vi "Result FGV.vi"(6 "Action(Get All Data)":T2=enum."Get All Data", 8 "error in":errorcluster, 11 "Result FGV Data In":T1) -> (0 "error out":errorcluster, 3 "Result FGV Data Out":T1)   [LabVIEW 2023, in "HardwareAbstractionLayer_LVOOP.lvlib" / "Report.lvclass"]
uses:
  Report.lvclass
  Control/Action FGV.ctl
  Control/Result FGV Data.ctl
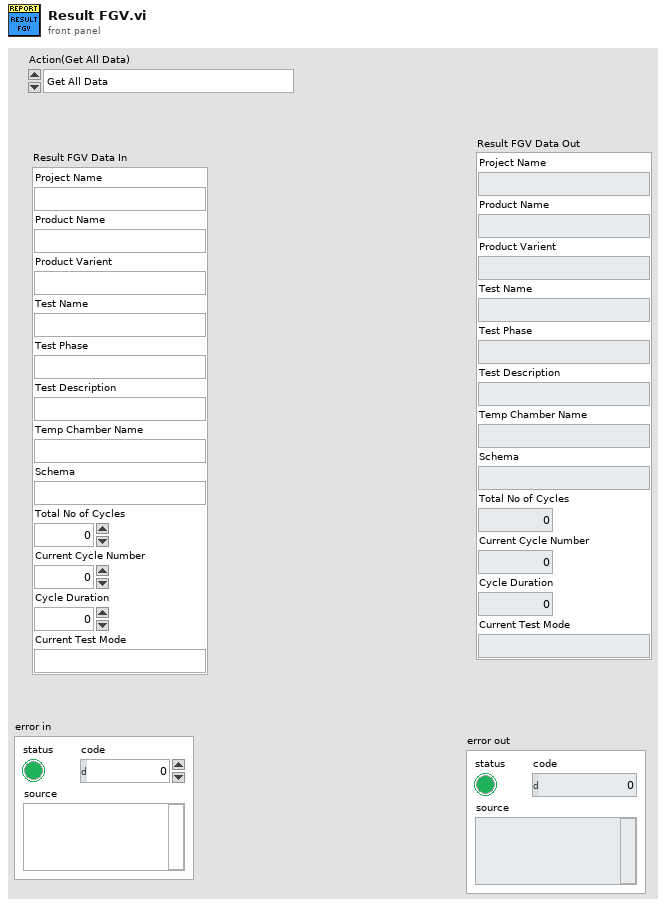
[diagram p1: front panel]
types:
  T1 = typedef "HardwareAbstractionLayer_LVOOP.lvlib/Report.lvclass/Result FGV Data.ctl" = cluster{"Project Name":string, "Product Name":string, "Product Varient":string, "Test Name":string, "Test Phase":string, "Test Description":string, "Temp Chamber Name":string, "Schema":string, "Total No of Cycles":u32, "Current Cycle Number":u32, "Cycle Duration":u32, "Current Test Mode":string}
  T2 = typedef "HardwareAbstractionLayer_LVOOP.lvlib/Report.lvclass/Action FGV.ctl" = enum16{"Init", "Set Project Name", "Set Product Name", "Set Product Varient", "Set Test Name", "Set Test Phase", "Set Test Description", "Set Temp Chamber Name", "Set Cycle Duration", "Set Current Cycle Number", "Set Schema", "Set Total No Of Cycle", "Set Current Test Mode", "Set All Data", "Get All Data"}
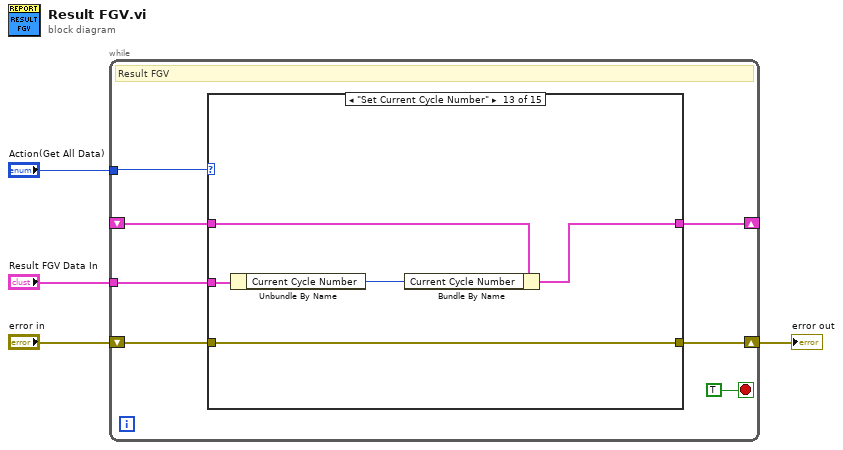
[diagram p0: block diagram]
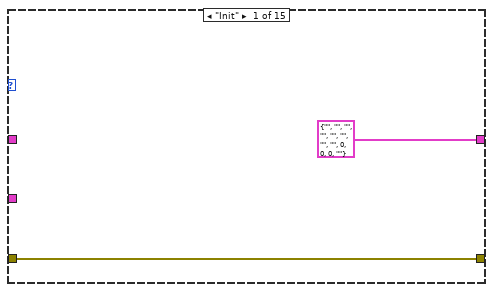
[diagram p2: hidden frame]
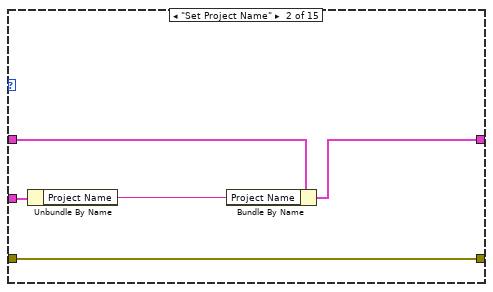
[diagram p3: hidden frame]
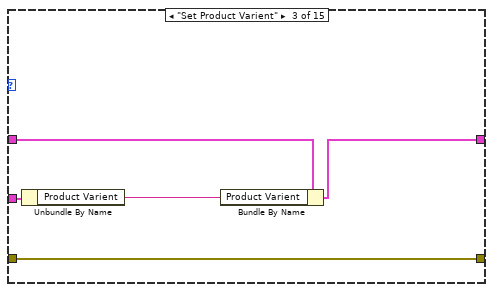
[diagram p4: hidden frame]
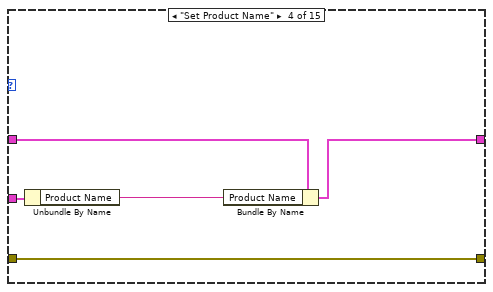
[diagram p5: hidden frame]
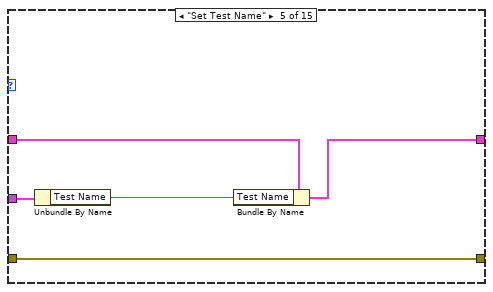
[diagram p6: hidden frame]
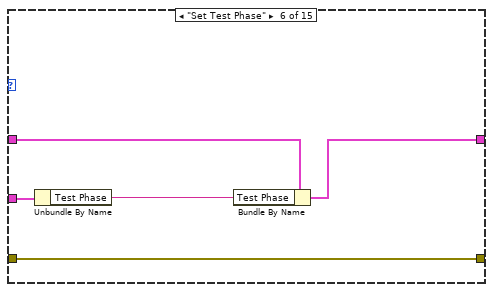
[diagram p7: hidden frame]
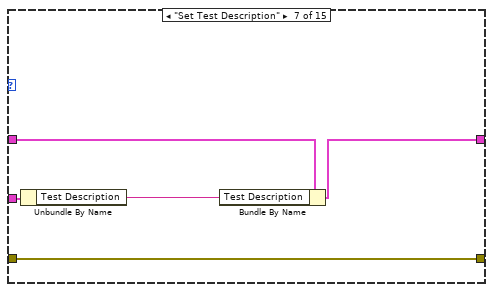
[diagram p8: hidden frame]
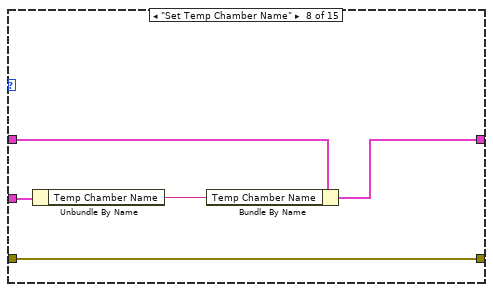
[diagram p9: hidden frame]
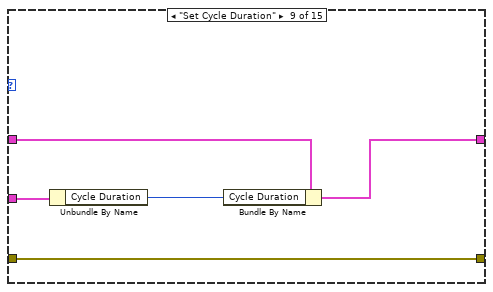
[diagram p10: hidden frame]
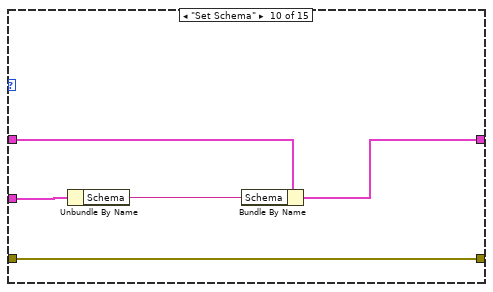
[diagram p11: hidden frame]
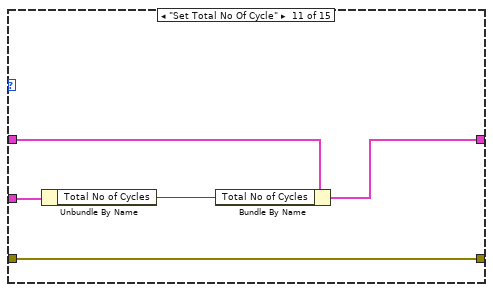
[diagram p12: hidden frame]
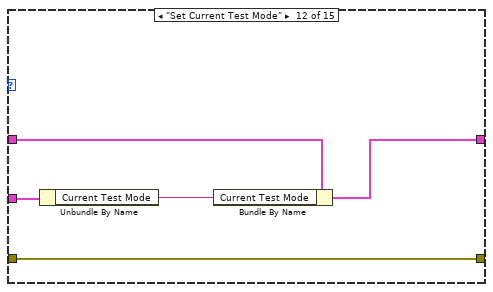
[diagram p13: hidden frame]
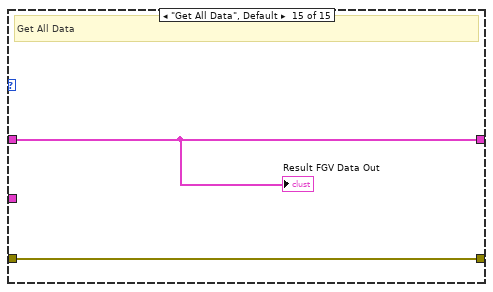
[diagram p15: hidden frame]
diagram:
  n1 = while {
    tunnel: "Action(Get All Data)" -> [w10]
    shift-right: [w8] -> w2
    shift-left: "error in" -> [w9]
    shift-right: [w6] -> _
    shift-left: _ -> [w7]
    tunnel: "Result FGV Data In" -> [w5]
    stop <- TRUE stop-if-true
    # "Result FGV"
    n2 = case shown="\"Set Current Cycle Number\"" w10 {
      tunnel: w9 -> [w13 w18 w23 w28 w33 w38 w43 w48 w53 w58 w63 w68 w73 w75 w77]
      tunnel: [w13 w18 w23 w28 w33 w38 w43 w48 w53 w58 w63 w68 w73 w75 w77] -> w8
      tunnel: w7 -> [_ w17 w22 w27 w32 w37 w42 w47 w52 w57 w62 w67 w72 _ w76]
      tunnel: [T1 {"Project Name"="", "Product Name"="", "Product Varient"="", "Test Name"="", "Test Phase"="", "Test Description"="", "Temp Chamber Name"="", "Schema"="", "Total No of Cycles"=0, "Current Cycle Number"=0, "Cycle Duration"=0, "Current Test Mode"=""} ("Result FGV Data") w16 w21 w26 w31 w36 w41 w46 w51 w56 w61 w66 w71 w74 w76] -> w6
      tunnel: w5 -> [_ w15 w20 w25 w30 w35 w40 w45 w50 w55 w60 w65 w70 w74 _]
      frame "Init" {
      }
      frame "Set Project Name" {
        n3 = Unbundle By Name(w15) -> ("Project Name"=w14:string)
        n4 = Bundle By Name(cluster=w17, "Project Name"=w14) -> (w16:T1)
      }
      frame "Set Product Varient" {
        n5 = Unbundle By Name(w20) -> ("Product Varient"=w19:string)
        n6 = Bundle By Name(cluster=w22, "Product Varient"=w19) -> (w21:T1)
      }
      frame "Set Product Name" {
        n7 = Unbundle By Name(w25) -> ("Product Name"=w24:string)
        n8 = Bundle By Name(cluster=w27, "Product Name"=w24) -> (w26:T1)
      }
      frame "Set Test Name" {
        n9 = Unbundle By Name(w30) -> ("Test Name"=w29:string)
        n10 = Bundle By Name(cluster=w32, "Test Name"=w29) -> (w31:T1)
      }
      frame "Set Test Phase" {
        n11 = Unbundle By Name(w35) -> ("Test Phase"=w34:string)
        n12 = Bundle By Name(cluster=w37, "Test Phase"=w34) -> (w36:T1)
      }
      frame "Set Test Description" {
        n13 = Unbundle By Name(w40) -> ("Test Description"=w39:string)
        n14 = Bundle By Name(cluster=w42, "Test Description"=w39) -> (w41:T1)
      }
      frame "Set Temp Chamber Name" {
        n15 = Unbundle By Name(w45) -> ("Temp Chamber Name"=w44:string)
        n16 = Bundle By Name(cluster=w47, "Temp Chamber Name"=w44) -> (w46:T1)
      }
      frame "Set Cycle Duration" {
        n17 = Unbundle By Name(w50) -> ("Cycle Duration"=w49:u32)
        n18 = Bundle By Name(cluster=w52, "Cycle Duration"=w49) -> (w51:T1)
      }
      frame "Set Schema" {
        n19 = Unbundle By Name(w55) -> ("Schema"=w54:string)
        n20 = Bundle By Name(cluster=w57, "Schema"=w54) -> (w56:T1)
      }
      frame "Set Total No Of Cycle" {
        n21 = Unbundle By Name(w60) -> ("Total No of Cycles"=w59:u32)
        n22 = Bundle By Name(cluster=w62, "Total No of Cycles"=w59) -> (w61:T1)
      }
      frame "Set Current Test Mode" {
        n23 = Unbundle By Name(w65) -> ("Current Test Mode"=w64:string)
        n24 = Bundle By Name(cluster=w67, "Current Test Mode"=w64) -> (w66:T1)
      }
      frame "Set Current Cycle Number" {
        n25 = Unbundle By Name(w70) -> ("Current Cycle Number"=w69:u32)
        n26 = Bundle By Name(cluster=w72, "Current Cycle Number"=w69) -> (w71:T1)
      }
      frame "Set All Data" {
      }
      frame "Get All Data", Default {
        # "Get All Data"
        "Result FGV Data Out" <- w76
      }
    }
  }
  "error out" <- w2
